vi "Save File Open Close Save References.vi"(6 "Save Data":string[](array[string]), 7 "Header Type":T3(ring), 8 "error in (no error)":errorcluster, 9 "New File?":bool, 10 "File Locations In":T1={"General Setup Paths"={"Calibration File Path"=path "", "DOE Capacity Path"=path "", "All Models Excel Sheet"=path "", "Network Model Location"=path "", "Data Folder Path"=path "", "DOE Backup"=path "", "Tool Base Path"=path "", "Configuration Path"=path "C:/Newfi Exe/Newfi Exe Locations.ini", "Appliance Prev Run Path"=path ""}, "Data File Paths"={"Data File Path"=path "", "Debug File Path"=path "", "Bus Log Path"=path "", "Current"=path "", "Summary"=path ""}, "New Summary Created"=FALSE, "Files Already Exist"=FALSE, "Check Location Interval (Second)"=0}, 11 "Byte Stream File in":refnum<file>) -> (0 "error out":errorcluster, 3 "Byte Stream File out":refnum<file>)   [LabVIEW 2016, in "Save File.lvlib"]
uses:
  Save File.lvlib
  File Setup (Public)/Type Definition/Save File DOE Data Save Filepaths.ctl
  File Setup.lvlib
  File Setup (Public)/Type Definition/Save File DOE File Path Control.ctl
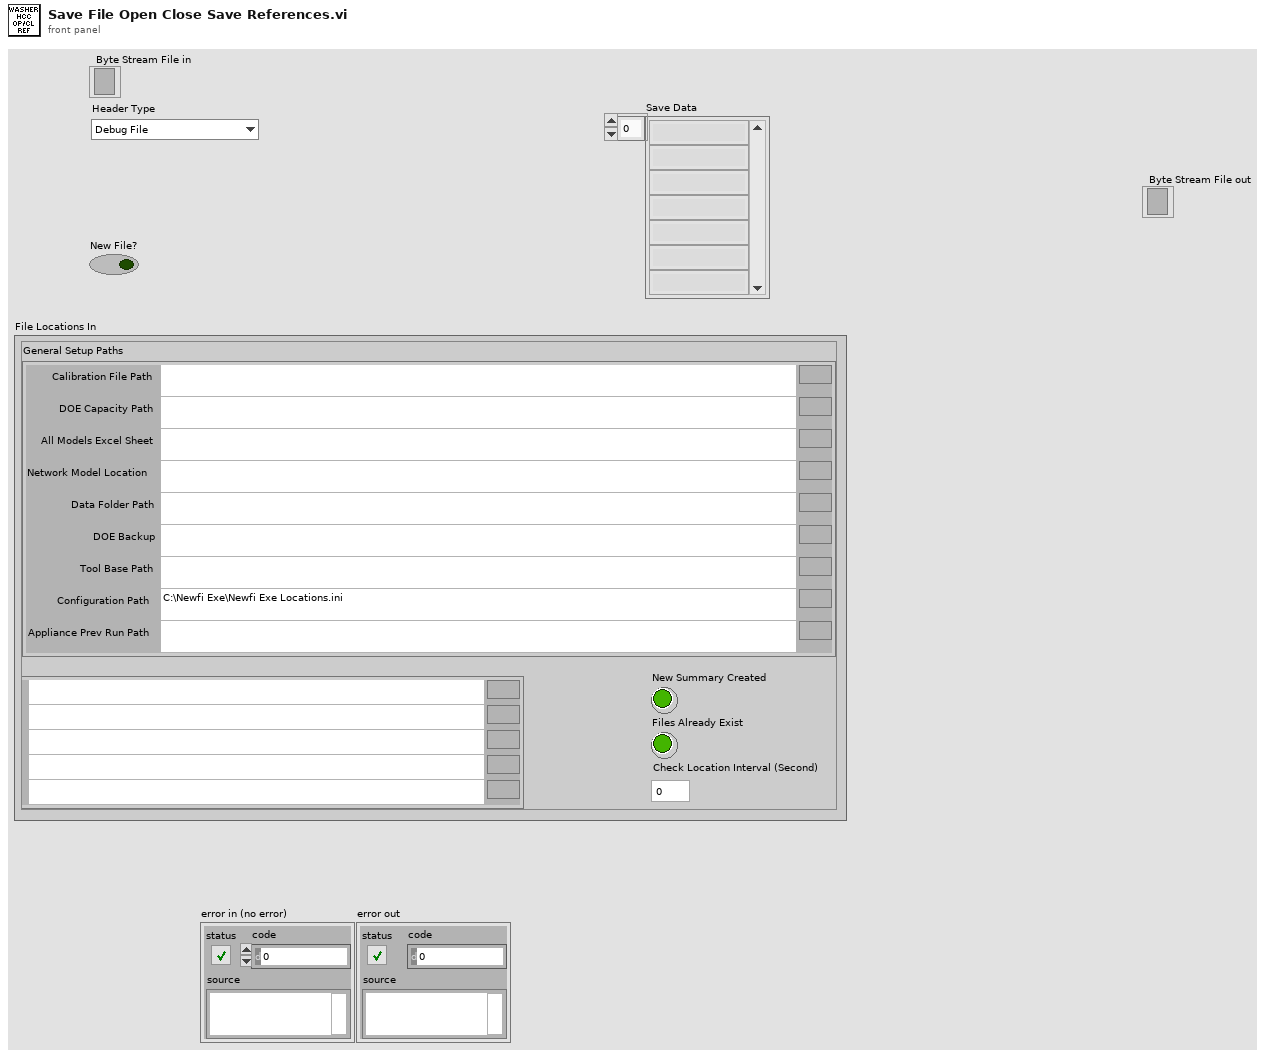
[diagram p1: front panel]
types:
  T1 = typedef "File Setup.lvlib/Save File DOE File Path Control.ctl" = cluster{"General Setup Paths":cluster{"Calibration File Path":path, "DOE Capacity Path":path, "All Models Excel Sheet":path, "Network Model Location":path, "Data Folder Path":path, "DOE Backup":path, "Tool Base Path":path, "Configuration Path":path, "Appliance Prev Run Path":path}, "Data File Paths":T2, "New Summary Created":bool, "Files Already Exist":bool, "Check Location Interval (Second)":i32}
  T2 = typedef "File Setup.lvlib/Save File DOE Data Save Filepaths.ctl" = cluster{"Data File Path":path, "Debug File Path":path, "Bus Log Path":path, "Current":path, "Summary":path}
  T3 = enum16{"Debug File", "Inverter File", "Current File", "Summary File", "Bus File"}
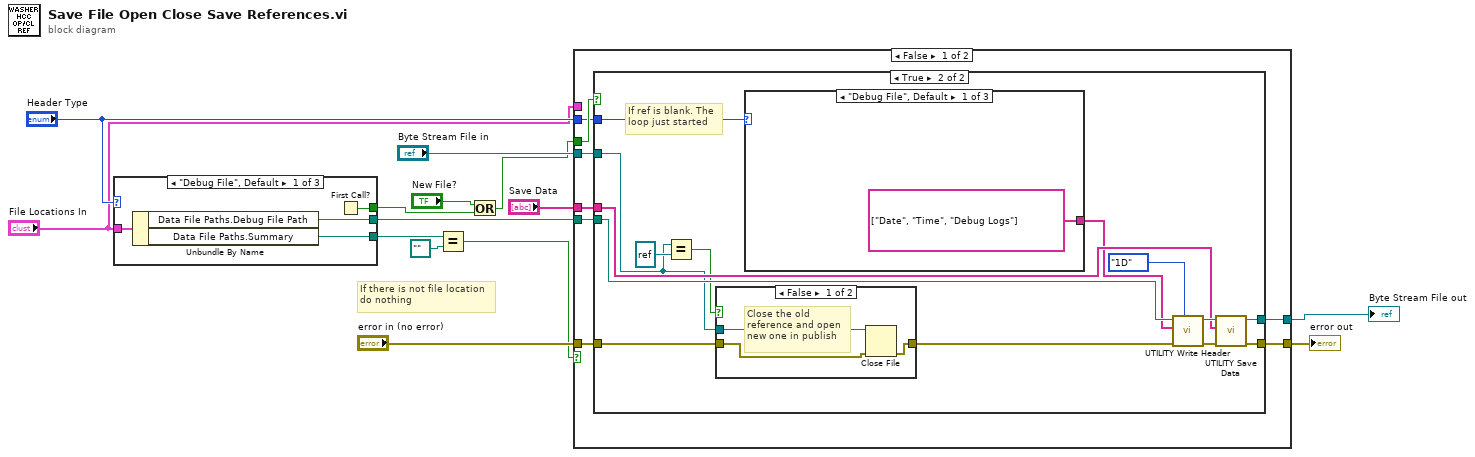
[diagram p0: block diagram]
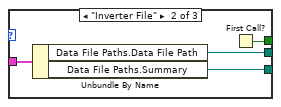
[diagram p2: hidden frame]
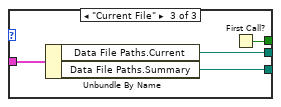
[diagram p3: hidden frame]
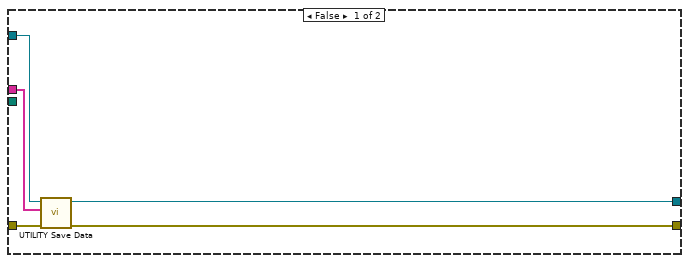
[diagram p4: hidden frame]
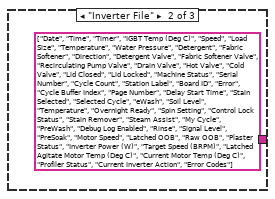
[diagram p5: hidden frame]
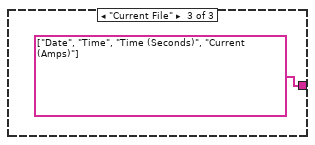
[diagram p6: hidden frame]
diagram:
  # "If there is not file location\ndo nothing"
  n1 = case shown="\"Debug File\", Default" "Header Type" {
    tunnel: [w17 w22 w24] -> w9
    tunnel: "File Locations In" -> [w18 w21 w26]
    tunnel: [w16 w20 w25] -> w7
    tunnel: [w15 w19 w23] -> w2
    frame "Debug File", Default {
      n2 = Unbundle By Name(w18) -> ("Data File Paths.Debug File Path"=w16:path, "Data File Paths.Summary"=w17:path)
      n3 = First Call?() -> (First Call?: T/F=w15:bool)
    }
    frame "Inverter File" {
      n4 = Unbundle By Name(w21) -> ("Data File Paths.Data File Path"=w20:path, "Data File Paths.Summary"=w22:path)
      n5 = First Call?() -> (First Call?: T/F=w19:bool)
    }
    frame "Current File" {
      n6 = Unbundle By Name(w26) -> ("Data File Paths.Current"=w25:path, "Data File Paths.Summary"=w24:path)
      n7 = First Call?() -> (First Call?: T/F=w23:bool)
    }
  }
  n8 = Equal?(x=w9, y=path "") -> (x = y?=w6:bool)
  n9 = Or(x="New File?", y=w2) -> (x .or. y?=w3:bool)
  n10 = case shown="False" w6 {
    tunnel: w3 -> [w34 _]
    tunnel: "Save Data" -> [w33 _]
    tunnel: "File Locations In" -> [_ _]
    tunnel: [w32 w62] -> w11
    tunnel: "Byte Stream File in" -> [w31 w62]
    tunnel: "error in (no error)" -> [w30 w61]
    tunnel: [w29 w61] -> w14
    tunnel: w7 -> [w28 _]
    tunnel: "Header Type" -> [w27 _]
    frame False {
      n11 = case shown="True" w34 {
        tunnel: w28 -> [_ w51]
        tunnel: w33 -> [w39 w50]
        tunnel: [w37 w49] -> w32
        tunnel: w31 -> [w38 w41]
        tunnel: w30 -> [w36 w42]
        tunnel: [w35 w45] -> w29
        tunnel: w27 -> [_ w44]
        frame False {
          n12 = call "UTILITY Save Data.vi"("error in"=w36, "Data"=w39, "refnum"=w38) -> ("error out"=w35:errorcluster, "refnum out"=w37:refnum<file>)  [unwired: 7 in]
        }
        frame True {
          # "If ref is blank. The\nloop just started"
          n13 = Equal?(x=w41, y=refnum<file> refnum ("Blank")) -> (x = y?=w47:bool)
          n14 = case shown="False" w47 {
            tunnel: w41 -> [w59 _]
            tunnel: w42 -> [w58 w60]
            tunnel: [w57 w60] -> w46
            frame False {
              # "Close the old\nreference and open\nnew one in publish"
              n15 = Close File(refnum=w59, error in=w58) -> (error out=w57:errorcluster)  [unwired: 1 out]
            }
            frame True {
            }
          }
          n16 = case shown="\"Debug File\", Default" w44 {
            tunnel: [string[] ["Date", "Time", "Debug Logs"] ("Debug Log Header") string[] ["Date", "Time", "Timer", "IGBT Temp (Deg C)", "Speed", "Load Size", "Temperature", "Water Pressure", "Detergent", "Fabric Softener", "Direction", "Detergent Valve", "Fabric Softener Valve", "Recirculating Pump Valve", "Drain Valve", "Hot Valve", "Cold Valve", "Lid Closed", "Lid Locked", "Machine Status", "Serial Number", "Cycle Count", "Station Label", "Board ID", "Error", "Cycle Buffer Index", "Page Number", "Delay Start Time", "Stain Selected", "Selected Cycle", "eWash", "Soil Level", "Temperature", "Overnight Ready", "Spin Setting", "Control Lock Status", "Stain Remover", "Steam Assist", "My Cycle", "PreWash", "Debug Log Enabled", "Rinse", "Signal Level", "PreSoak", "Motor Speed", "Latched OOB", "Raw OOB", "Plaster Status", "Inverter Power (W)", "Target Speed (BRPM)", "Latched Agitate Motor Temp (Deg C)", "Current Motor Temp (Deg C)", "Profiler Status", "Current Inverter Action", "Error Codes"] ("Inv and MC Header") string[] ["Date", "Time", "Time (Seconds)", "Current (Amps)"] ("Current Header")] -> w40
            frame "Debug File", Default {
            }
            frame "Inverter File" {
            }
            frame "Current File" {
            }
          }
          n17 = call "UTILITY Write Header.vi"("Array Type"=enum16{"1D", "2D"}."1D", "error in (no error)"=w46, "Headers"=w40, "File Path Control"=w51) -> ("error out"=w53:errorcluster, "Byte Stream File out"=w52:refnum<file>)  [unwired: 6 in]
          n18 = call "UTILITY Save Data.vi"("error in"=w53, "Data"=w50, "refnum"=w52) -> ("error out"=w45:errorcluster, "refnum out"=w49:refnum<file>)  [unwired: 7 in]
        }
      }
    }
    frame True {
    }
  }
  "error out" <- w14
  "Byte Stream File out" <- w11
